vi "Send Star Trigger.vi"(8 "error in (no error)":errorcluster, 11 "VISA resource name":refnum<visa-resource-name>) -> (0 "error out":errorcluster, 3 "VISA resource name out":refnum<visa-resource-name>)   [LabVIEW 2010, in "Agilent U2722.lvlib"]
doc: "Send a star trigger to the slave components in the same chassis. Call <B>Configure Synchronous Simultaneous Interface VI</B> to set the slave components. \n\n<B>Note:</B>\n\nThis VI has been obsoleted from the driver and is included for compatibility with existing applications."
uses:
  Agilent U2722.lvlib
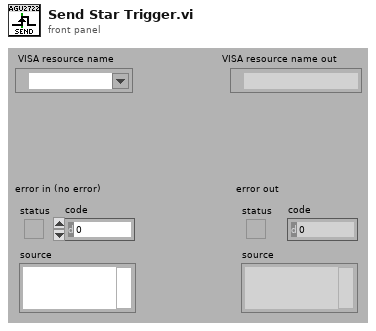
[diagram p1: front panel]
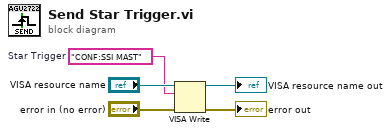
[diagram p0: block diagram]
diagram:
  w3 = "CONF:SSI MAST"  # Star Trigger
  n1 = VISA Write(VISA resource name="VISA resource name", write buffer=w3, error in (no error)="error in (no error)") -> (VISA resource name out=→"VISA resource name out":refnum<visa-resource-name>, error out=→"error out":errorcluster)  [unwired: 1 out]
